vi "BEEPTIT.vi"(8 "error in":errorcluster) -> (0 "error out":errorcluster)   [LabVIEW 2009]
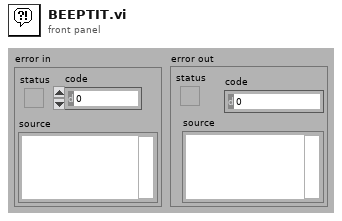
[diagram p1: front panel]
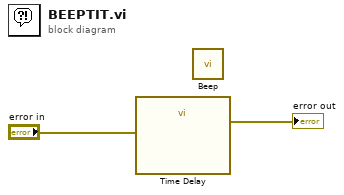
[diagram p0: block diagram]
diagram:
  n1 = call "Time Delay"("error in (no error)"="error in") -> ("error out"=→"error out":errorcluster)  [unwired: 10 in]
  n2 = call <vilib>:"Beep.vi"() -> ()  [unwired: 12 in]
